vi "GenAcqSound.vi"() -> ()   [LabVIEW 2017]
uses:
  <vilib>/sound2/lvsound2.llb/Sound Data Format.ctl
  <vilib>/sound2/lvsound2.llb/Sampling Mode.ctl
  <vilib>/sound2/lvsound2.llb/Sound Output Write (DBL Single).vi
  <vilib>/sound2/lvsound2.llb/Sound Input Read (DBL).vi
  <vilib>/measure/matone.llb/Extract Single Tone Information N Chan.vi
  <vilib>/measure/NI_MABase.lvlib
  <vilib>/measure/NI_MAPro.lvlib
panel:
  out "detected frequencies":dbl[](array[numeric]) format="%.2p"
  in  "Acq # of samples/ch":i32=10000
  out "Acq Audio":waveform(dbl)[](graph)
  in  "Signal":string(combo)
  in  "stop":bool
  out "Gen Audio":waveform(dbl)(graph)
  in  "amplitude":dbl(slide)=1.0 scale=0.0..3.0
  in  "frequency":dbl(knob)=10.0 scale=0.0..1000.0
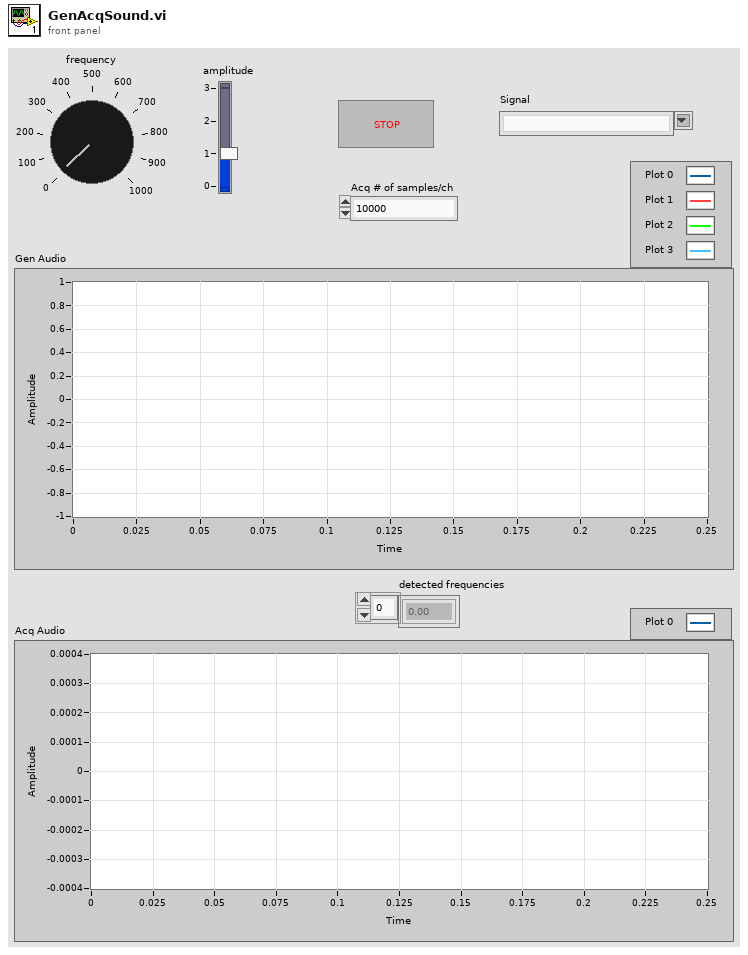
[diagram p1: front panel]
types:
  T1 = typedef "Sampling Mode.ctl" = i32
  T2 = typedef "Sound Data Format.ctl" = cluster{"sample rate (S/s)":dbl, "number of channels":i32, "bits per sample":i32}
  T3 = typedef "Sound Input Task ID.ctl" = u32
  T4 = typedef "Sound Output Task ID.ctl" = u32
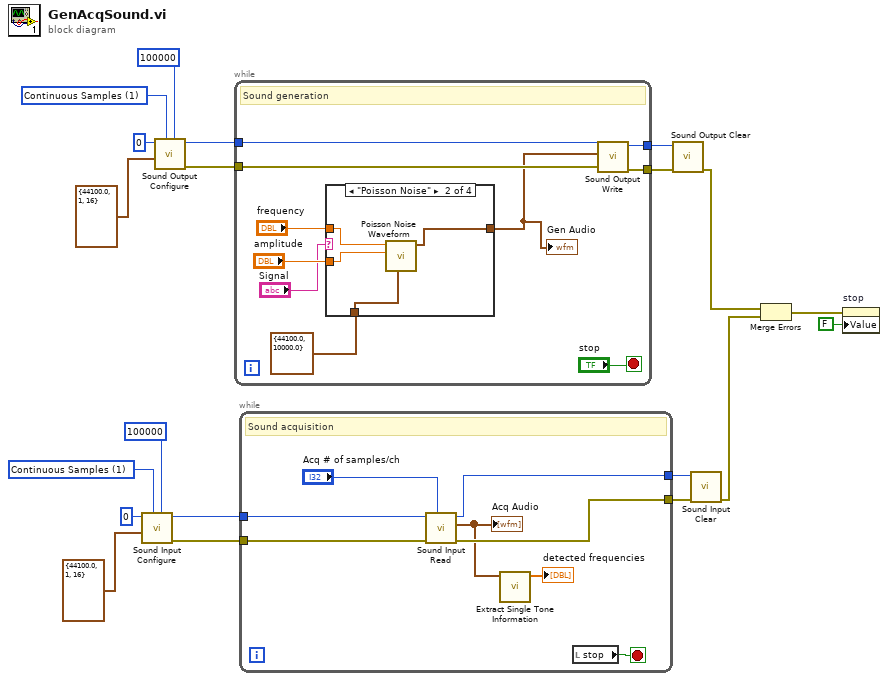
[diagram p0: block diagram]
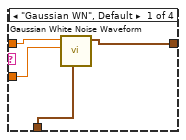
[diagram p2: hidden frame]
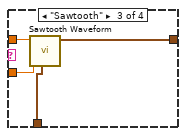
[diagram p3: hidden frame]
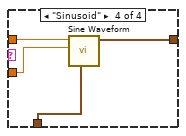
[diagram p4: hidden frame]
diagram:
  w9 = T1 1 items=["Finite Samples", "Continuous Samples"] ("sample mode")
  w17 = T1 1 items=["Finite Samples", "Continuous Samples"] ("sample mode")
  n1 = call <vilib>:"Sound Input Configure.vi"("number of samples/ch"=100000, "sample mode"=w9, "sound format"=T2 {"sample rate (S/s)"=44100.0, "number of channels"=1, "bits per sample"=16}, "device ID"=u32 0) -> ("error out"=w7:errorcluster, "task ID"=w8:T3)  [unwired: 6 in]
  n2 = call <vilib>:"Sound Output Configure.vi"("number of samples/ch"=100000, "sample mode"=w17, "sound format"=T2 {"sample rate (S/s)"=44100.0, "number of channels"=1, "bits per sample"=16}, "device ID"=u32 0) -> ("error out"=w16:errorcluster, "task ID"=w15:T4)  [unwired: 6 in]
  n3 = while {
    tunnel: w16 -> [w29]
    tunnel: w15 -> [w30]
    tunnel: [w26] -> w14
    tunnel: [w25] -> w13
    stop <- "stop" stop-if-true
    # "Sound generation"
    n4 = case shown="\"Poisson Noise\"" "Signal" {
      tunnel: "frequency" -> [w33 w36 w42 w46]
      tunnel: "amplitude" -> [w32 w37 w41 w45]
      tunnel: [w31 w35 w40 w43] -> w21
      tunnel: cluster{"Fs":dbl, "#s":dbl} {"Fs"=44100.0, "#s"=10000.0} ("sampling info") -> [w34 w38 w39 w44]
      frame "Gaussian WN", Default {
        n5 = call <vilib>:"Gaussian White Noise Waveform.vi"("sampling info"=w34, "seed"=w32, "standard deviation"=w33) -> ("signal out"=w31:waveform(dbl))  [unwired: 7 in, 1 out]
      }
      frame "Poisson Noise" {
        n6 = call <vilib>:"Poisson Noise Waveform.vi"("sampling info"=w38, "seed"=w37, "mean"=w36) -> ("signal out"=w35:waveform(dbl))  [unwired: 7 in, 1 out]
      }
      frame "Sawtooth" {
        n7 = call <vilib>:"Sawtooth Waveform.vi"("sampling info"=w39, "amplitude"=w41, "frequency"=w42) -> ("signal out"=w40:waveform(dbl))  [unwired: 7 in, 1 out]
      }
      frame "Sinusoid" {
        n8 = call <vilib>:"Sine Waveform.vi"("sampling info"=w44, "amplitude"=w45, "frequency"=w46) -> ("signal out"=w43:waveform(dbl))  [unwired: 7 in, 1 out]
      }
    }
    "Gen Audio" <- w21
    n9 = call-poly <vilib>:"Sound Output Write.vi"("error in (no error)"=w29, "data"=w21, "task ID"=w30) -> ("error out"=w25:errorcluster, "task ID out"=w26:T4)  [unwired: 7 in]
  }
  n10 = while {
    tunnel: w8 -> [w53]
    tunnel: w7 -> [w52]
    tunnel: [w51] -> w6
    tunnel: [w50] -> w5
    stop <- w54 stop-if-true
    # "Sound acquisition"
    n11 = call-poly <vilib>:"Sound Input Read.vi"("number of samples/ch"="Acq # of samples/ch", "error in (no error)"=w52, "task ID"=w53) -> ("error out"=w51:errorcluster, "data"=w48:waveform(dbl)[], "task ID out"=w50:T3)  [unwired: 6 in]
    "Acq Audio" <- w48
    n12 = call-poly <vilib>:"Extract Single Tone Information.vi"("time signals in"=w48) -> ("detected frequencies"=→"detected frequencies":dbl[])  [unwired: 5 in, 5 out]
    n13 = local read "stop"() -> (w54:bool)
  }
  n14 = call <vilib>:"Sound Output Clear.vi"("error in (no error)"=w13, "task ID"=w14) -> ("error out"=w3:errorcluster)  [unwired: 9 in]
  n15 = call <vilib>:"Sound Input Clear.vi"("error in (no error)"=w6, "task ID"=w5) -> ("error out"=w4:errorcluster)  [unwired: 9 in]
  n16 = Merge Errors(w3, w4) -> (w2:errorcluster)
  n17 = property on="stop" class="Bool (strict)"(error in=w2, "Value"=FALSE ("stop")) -> ()  [unwired: 1 in, 2 out]
